vi "Write Initial State.vi"(10 "Initial State":refnum<class "state.lvclass">) -> (2 "Unknown State":refnum<class "state.lvclass">)   [LabVIEW 2020, in "eos.lvlib" / "unknown.lvclass"]
uses:
  unknown.lvclass
  C:/Projects/LVOS/EngineeringOS/source/classes/states/unknown/unknown.lvclass
  C:/Projects/LVOS/EngineeringOS/source/interfaces/state/state.lvclass
  interfaces/state/state.lvclass
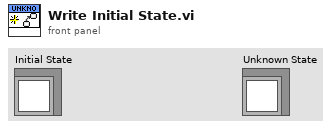
[diagram p1: front panel]
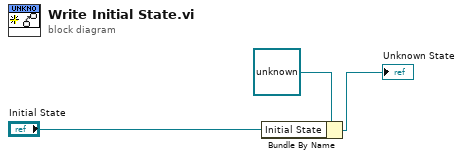
[diagram p0: block diagram]
diagram:
  n1 = Bundle By Name(cluster=refnum<class "unknown.lvclass"> refnum ("unknown in"), "Initial State"="Initial State") -> (→"Unknown State":refnum<class "unknown.lvclass">)
